vi "data to xy cluster.vi"(10 "Index":i32, 11 "Combined Data":dbl[][](array[numeric])) -> (3 "input cluster":cluster{"Time":dbl[], "State 1":dbl[]})   [LabVIEW 2025, in "Dynamic-System.lvclass"]
uses:
  Dynamic-System.lvclass
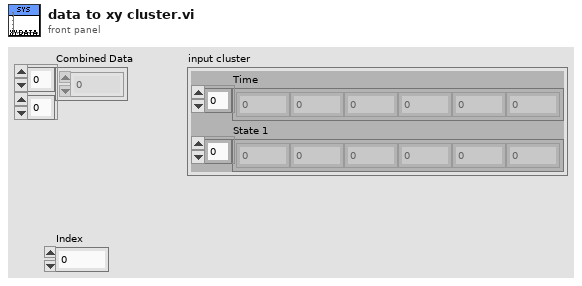
[diagram p1: front panel]
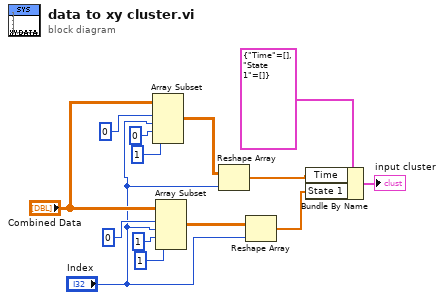
[diagram p0: block diagram]
diagram:
  n1 = Array Subset(array="Combined Data", index (row)=0 ("index"), length (row)="Index", index (col)=0 ("index"), length (col)=1 ("length")) -> (w2:dbl[][])
  n2 = Array Subset(array="Combined Data", index (row)=0 ("index"), length (row)="Index", index (col)=1 ("index"), length (col)=1 ("length")) -> (w13:dbl[][])
  n3 = Reshape Array(w2, "Index") -> (w1:dbl[])
  n4 = Reshape Array(w13, "Index") -> (w12:dbl[])
  n5 = Bundle By Name(cluster=cluster{"Time":dbl[], "State 1":dbl[]} {"Time"=[], "State 1"=[]} ("input cluster"), "Time"=w1, "State 1"=w12) -> (→"input cluster":cluster{"Time":dbl[], "State 1":dbl[]})
